vi "Find All Uses.Dialog.vi"(11 "found":refnum<vi>[](array[refnum])) -> ()   [LabVIEW 2020]
doc: "Use this template to create a dialog box with event handling."
panel:
  in  "Copy to Clipboard":bool
  in  "Uses of the element":i32(listbox)
  in  "OK":bool
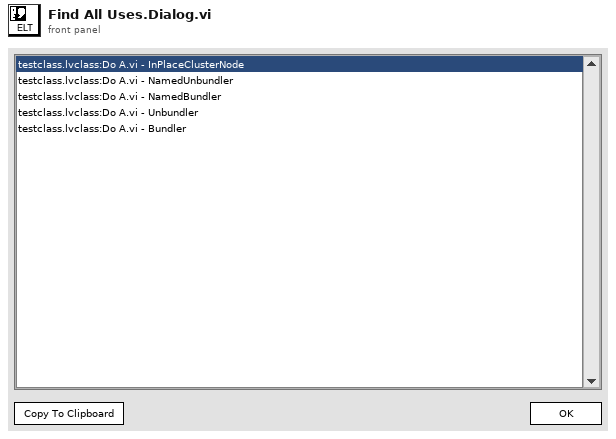
[diagram p1: front panel]
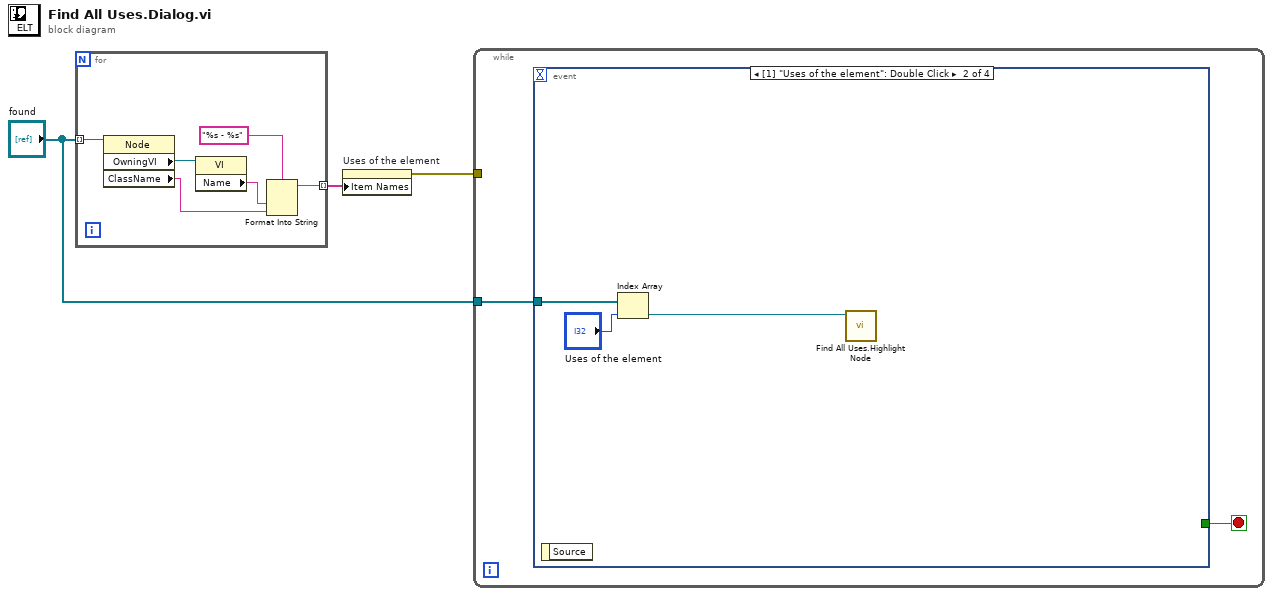
[diagram p0: block diagram]
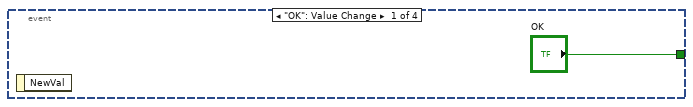
[diagram p2: hidden frame]
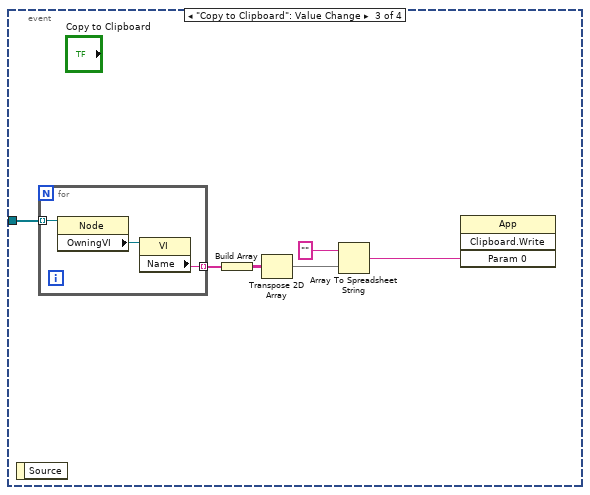
[diagram p3: hidden frame]
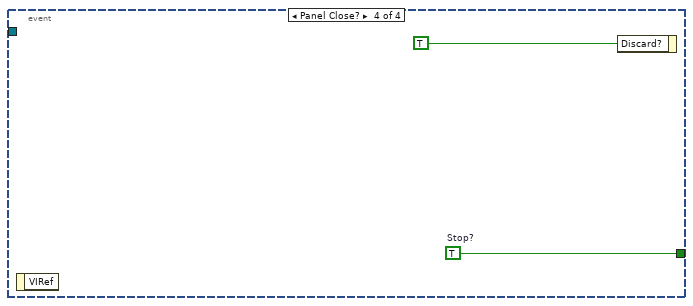
[diagram p4: hidden frame]
diagram:
  n1 = for {
    tunnel: "found" -> [w9] mode=indexing
    tunnel: [w4] -> w3 mode=indexing
    n2 = property class="Node"(reference=w9) -> ("OwningVI"=w8:refnum<vi>, "ClassName"=w5:string)  [unwired: 1 in, 2 out]
    n3 = property class="VI"(reference=w8) -> ("Name"=w7:string)  [unwired: 1 in, 2 out]
    n4 = Format Into String(format string="%s - %s", w7, w5) -> (resulting string=w4:string)  [unwired: 2 in, 1 out]
  }
  n5 = property on="Uses of the element" class="LstBox (strict)"("Item Names"=w3) -> (error out=w2:errorcluster)  [unwired: 2 in, 1 out]
  n6 = while {
    tunnel: w2 -> [_]
    tunnel: "found" -> [w10]
    stop <- w11 stop-if-true
    n7 = event shown="[1] \"Uses of the element\": Double Click" {
      selector: _ -> [_ _ _ _]
      dyn-events: _ -> [_ _ _ _]
      timeout: _ -> [_ _ _ _]
      tunnel: ["OK" _ _ w25] -> w11
      tunnel: w10 -> [_ w15 w21 _]
      event "OK": Value Change {
        n8 = event-data() -> ()  [unwired: 1 in, 1 out]
      }
      event "Uses of the element": Double Click {
        n9 = event-data() -> ()  [unwired: 1 in, 1 out]
        n10 = Index Array(array=w15, index="Uses of the element") -> (element=w13:refnum<vi>)
        n11 = call "Find All Uses.Highlight Node.vi"("Node in"=w13) -> ()  [unwired: 11 in]
      }
      event "Copy to Clipboard": Value Change {
        n12 = event-data() -> ()  [unwired: 1 in, 1 out]
        n13 = for {
          tunnel: w21 -> [w23] mode=indexing
          tunnel: [w22] -> w20 mode=indexing
          n14 = property class="Node"(reference=w23) -> ("OwningVI"=w24:refnum<vi>)  [unwired: 1 in, 2 out]
          n15 = property class="VI"(reference=w24) -> ("Name"=w22:string)  [unwired: 1 in, 2 out]
        }
        n16 = Build Array(w20) -> (w19:string[][])
        n17 = Transpose 2D Array(2D array=w19) -> (transposed array=w18:string[][])
        n18 = Array To Spreadsheet String(array=w18, 3:"" ("format string")) -> (spreadsheet string=w17:string)  [unwired: 1 in]
        n19 = invoke class="App" method="Clipboard.Write"("Param 0"=w17) -> ()  [unwired: 3 in, 4 out]
      }
      event Panel Close? {
        w25 = TRUE  # Stop?
        n20 = event-data() -> ()  [unwired: 1 in, 1 out]
        n21 = event-data("Discard?"=TRUE) -> ()  [unwired: 1 in, 1 out]
      }
    }
  }
